vi "AVS_PollScan.vi"(9 "a_hDevice":i32) -> (3 "Output Value":i32)   [LabVIEW 2013, in "AvaSpec.lvlib" / "Avantes Spectrometer Functions.lvlib"]
uses:
  Avantes Spectrometer Functions.lvlib
  AS5216.dll
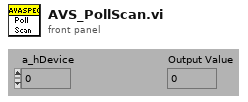
[diagram p1: front panel]
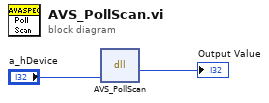
[diagram p0: block diagram]
diagram:
  n1 = dll-call lib="C:/Users/dhstuart/Dropbox/CLTC/avantesSpectrometer/Libraries/AS-5216-DLL/polling_mc/AS5216.dll" fn="AVS_PollScan"("a_hDevice"="a_hDevice") -> (→"Output Value":i32)  [unwired: 4 in, 2 out]
